vi "init.vi"(8 "error in (no error)":errorcluster, 11 "Cafe in":refnum<class "Cafe.lvclass">) -> (0 "error out":errorcluster, 3 "Cafe out":refnum<class "Cafe.lvclass">)   [LabVIEW 2020, in "Cafe.lvlib" / "Cafe.lvclass"]
uses:
  Cafe.lvclass
  C:/Program Files (x86)/National Instruments/LabVIEW 2020/vi.lib/ActorFramework/Actor/Actor.lvclass
  <vilib>/ActorFramework/Actor/Actor.lvclass/Actor.ctl
  Cafe.lvclass/Cafe.ctl
  UI Actor Messages/Write Path Msg/Write Path Msg.lvclass/Write Path Msg.ctl
  <vilib>/ActorFramework/Message Enqueuer/Message Enqueuer.lvclass/Message Enqueuer.ctl
  <vilib>/ActorFramework/Message Enqueuer/Enqueue.vi
  UI Actor Messages/Write Path Msg/Write Path Msg.lvclass
  C:/Program Files (x86)/National Instruments/LabVIEW 2020/vi.lib/ActorFramework/Message/Message.lvclass
  <vilib>/ActorFramework/Message Priority Queue/Priority Enqueue.vi
  <vilib>/ActorFramework/Actor/Actor.lvclass
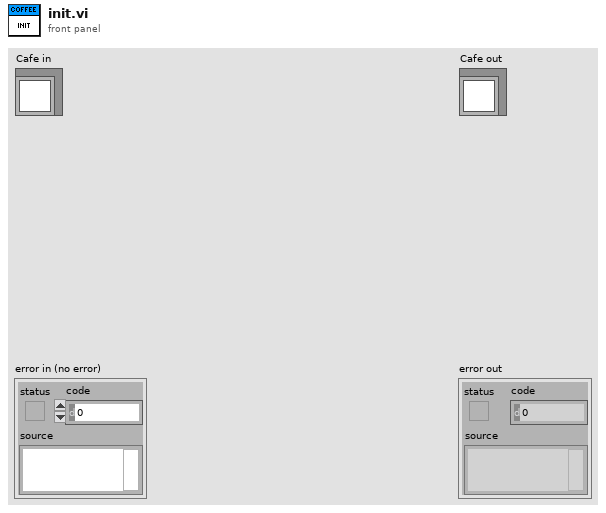
[diagram p1: front panel]
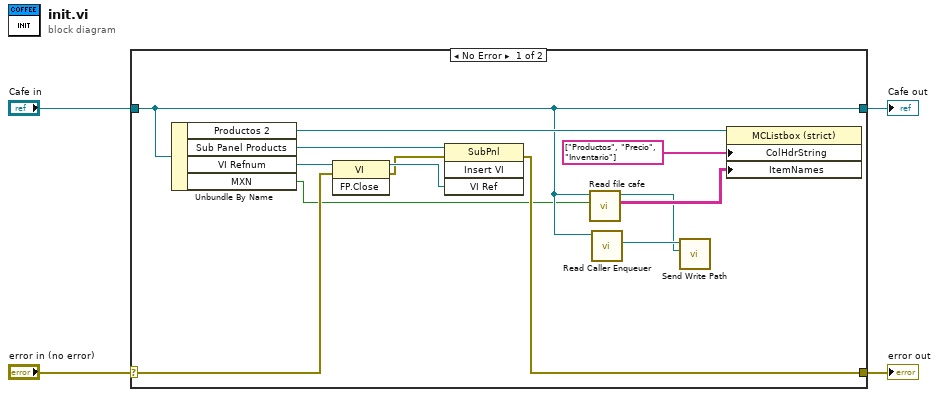
[diagram p0: block diagram]
diagram:
  n1 = case shown="No Error" "error in (no error)" {
    selector: "error in (no error)" -> [w13 w19]
    tunnel: [w12 w19] -> w3
    tunnel: [w9 w18] -> w1
    tunnel: "Cafe in" -> [w9 w18]
    frame No Error {
      n2 = Unbundle By Name(w9) -> ("Productos 2"=w11:refnum<vi>, "Sub Panel Products"=w17:refnum<vi>, "VI Refnum"=w16:refnum<vi>, "MXN"=w5:bool)
      n3 = invoke class="VI" method="FP.Close"(reference=w16, error in=w13) -> (reference out=w15:refnum<vi>, error out=w14:errorcluster)  [unwired: 1 in, 1 out]
      n4 = invoke class="SubPnl" method="Insert VI"(reference=w17, error in=w14, "VI Ref"=w15) -> (error out=w12:errorcluster)  [unwired: 1 in, 3 out]
      n5 = call "Read file cafe.vi"("MXN"=w5, "Cafe in"=w9) -> ("Item Names"=w8:string[][], "path"=w6:path)  [unwired: 8 in]
      n6 = call <vilib>:"Read Caller Enqueuer.vi"("Actor"=w9) -> ("Caller Enqueuer"=w7:refnum<class "Message Enqueuer.lvclass">)  [unwired: 10 in]
      n7 = call "Send Write Path.vi"("Path"=w6, "Message Enqueuer"=w7) -> ()  [unwired: 8 in, 2 out]
      n8 = property class="MCListbox (strict)"(reference=w11, "ColHdrString"=string[] ["Productos", "Precio", "Inventario"] ("Column Header Strings[]"), "ItemNames"=w8) -> ()  [unwired: 1 in, 2 out]
    }
    frame Error {
    }
  }
  "error out" <- w3
  "Cafe out" <- w1
